vi "Calibracion.vi"() -> ()   [LabVIEW 2013]
uses:
  Multicard III_Hardware_Module Control.ctl
  P2022 TB INCAR GLOBALES.vi
panel:
  out "Waveform Chart":dbl(graph)
  in  "BorraGrafica":bool
  out "Estado":bool
  out "error out":errorcluster
  in  "error in (no error)":errorcluster
  out "Peso de calibración":string
  out "Lectura A/D ?":i32
  out "Termopar":string
  in  "CambioNP":bool
  out "Núm. promedios":i32 max=255 step=1
  out "Lectura A/D Cero":i32
  out "Lectura A/D Span":i32
  out "Lectura A/D":i32
  in  "Help":bool
  out "Peso (mg)":dbl format="%.3f"
  in  "Exit":bool
  in  "Calibrate":bool
  in  "Zero":bool
  out "Temperatura (C)":dbl format="%.1f"
  # "Calibración termobalanza"
  # "Termobalanza"
  # "Lecturas de calibración A/D"
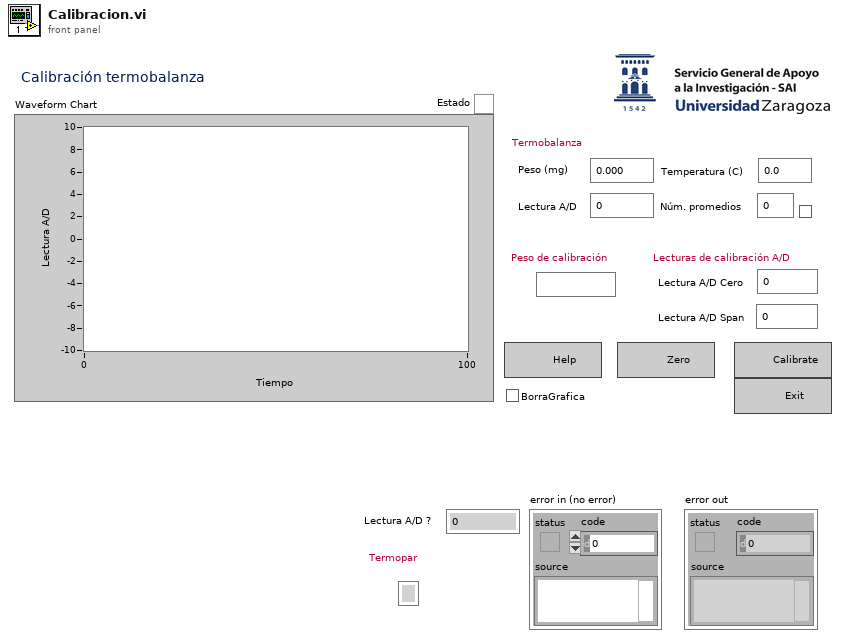
[diagram p1: front panel]
types:
  T1 = typedef "P2018 Com Control.ctl" = cluster{"Flujo_1":refnum<visa-resource-name>, "Brk1":bool, "Flujo_2":refnum<visa-resource-name>, "Brk2":bool, "Flujo_3":refnum<visa-resource-name>, "Brk3":bool, "Flujo_4":refnum<visa-resource-name>, "Brk4":bool, "Eurothe":refnum<visa-resource-name>, "Eurot":bool, "Balanza":refnum<visa-resource-name>, "Bal":bool, "eValPos":refnum<visa-resource-name>, "eVal":bool, "flowbus":refnum<visa-resource-name>, "fb":bool}
  T2 = typedef "Multicard III_Hardware_Module Control.ctl" = enum16{"Initialize", "Cero", "Span", "Read ugr", "Read mgr", "Read A/D", "Read T", "Number readings", "Thermocouple type", "Status", "Shutdown"}
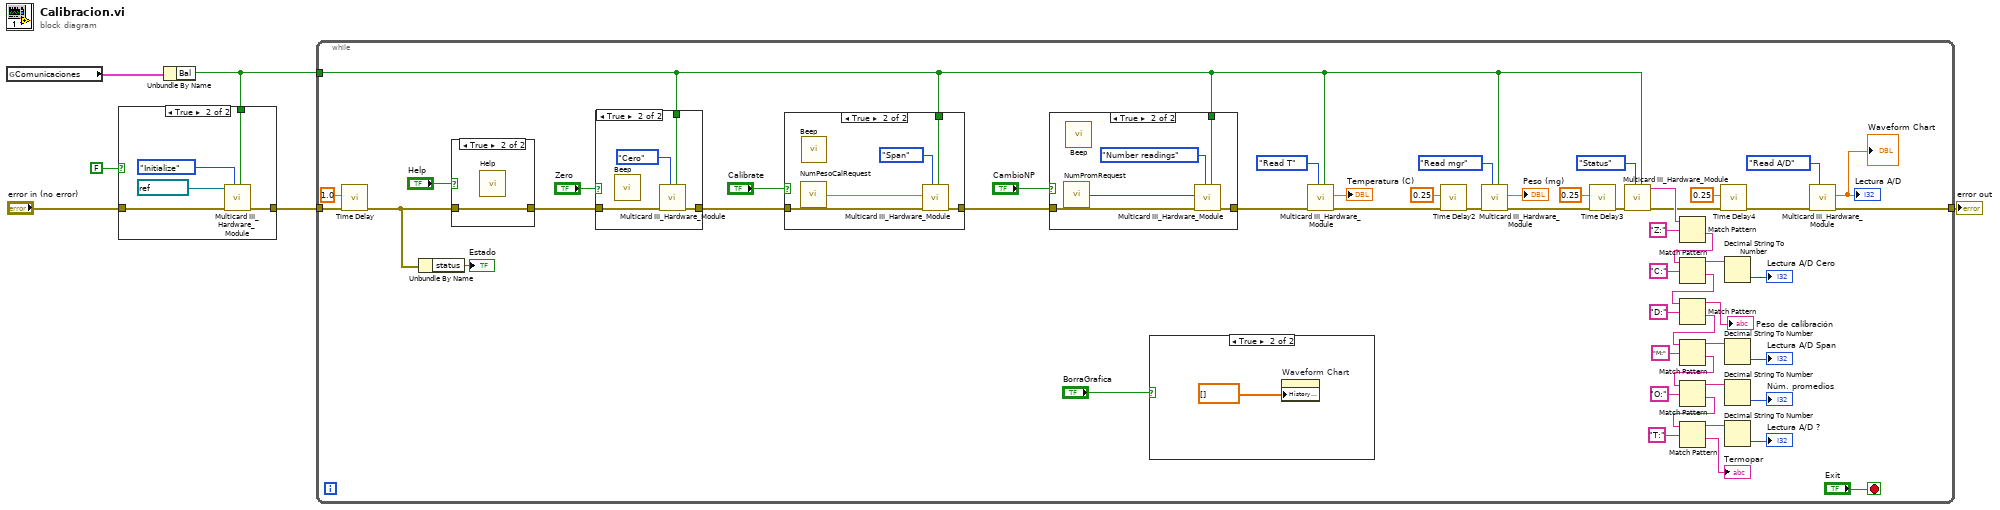
[diagram p0: block diagram]
diagram:
  n1 = global read "P2022 TB INCAR GLOBALES.vi" "Comunicaciones"() -> (w2:T1)
  n2 = Unbundle By Name(w2) -> ("Bal"=w1:bool)
  n3 = case shown="True" FALSE {
    tunnel: "error in (no error)" -> [w7 w11]
    tunnel: [w7 w10] -> w4
    tunnel: w1 -> [_ w8]
    frame False {
    }
    frame True {
      n4 = call "Multicard III_Hardware_Module.vi"("Multicard (T:Enable)"=w8, "Command"=Multicard_III_Hardware_Module_Control."Initialize", "error in (no error)"=w11, "VISA resource name"=refnum<visa-resource-name> "COM4") -> ("error out"=w10:errorcluster)  [unwired: 4 in, 3 out]
    }
  }
  n5 = while {
    tunnel: [w36] -> w6
    tunnel: w4 -> [w27]
    tunnel: w1 -> [w14]
    stop <- "Exit" stop-if-true
    n6 = call "Time Delay"("error in (no error)"=w27, "Delay Time (s)"=1.0) -> ("error out"=w26:errorcluster)  [unwired: 9 in]
    n7 = Unbundle By Name(w26) -> ("status"=→"Estado":bool)
    n8 = case shown="True" "Help" {
      tunnel: w26 -> [w80 w81]
      tunnel: [w80 w81] -> w35
      frame False {
      }
      frame True {
        n9 = call "Help.vi"() -> ()  [unwired: 1 in]
      }
    }
    n10 = case shown="True" "Zero" {
      tunnel: w35 -> [w82 w85]
      tunnel: [w82 w84] -> w33
      tunnel: w14 -> [_ w83]
      frame False {
      }
      frame True {
        n11 = call <vilib>:"Beep.vi"() -> ()  [unwired: 12 in]
        n12 = call "Multicard III_Hardware_Module.vi"("Multicard (T:Enable)"=w83, "Command"=Multicard_III_Hardware_Module_Control."Cero", "error in (no error)"=w85) -> ("error out"=w84:errorcluster)  [unwired: 5 in, 3 out]
      }
    }
    n13 = case shown="True" "Calibrate" {
      tunnel: w33 -> [w74 w76]
      tunnel: [w74 w78] -> w31
      tunnel: w14 -> [_ w75]
      frame False {
      }
      frame True {
        n14 = call "NumPesoCalRequest.vi"() -> ("NumProm"=w77:dbl)  [unwired: 1 in]
        n15 = call <vilib>:"Beep.vi"() -> ()  [unwired: 12 in]
        n16 = call "Multicard III_Hardware_Module.vi"("Multicard (T:Enable)"=w75, "Command"=Multicard_III_Hardware_Module_Control."Span", "error in (no error)"=w76, "Input Value"=w77) -> ("error out"=w78:errorcluster)  [unwired: 4 in, 3 out]
      }
    }
    n17 = case shown="True" "CambioNP" {
      tunnel: w31 -> [w68 w70]
      tunnel: [w68 w72] -> w30
      tunnel: w14 -> [_ w69]
      frame False {
      }
      frame True {
        n18 = call "NumPromRequest.vi"() -> ("NumProm"=w71:u8)  [unwired: 1 in]
        n19 = call <vilib>:"Beep.vi"() -> ()  [unwired: 12 in]
        n20 = call "Multicard III_Hardware_Module.vi"("Multicard (T:Enable)"=w69, "Command"=Multicard_III_Hardware_Module_Control."Number readings", "error in (no error)"=w70, "Input Value"=w71) -> ("error out"=w72:errorcluster)  [unwired: 4 in, 3 out]
      }
    }
    n21 = case shown="True" "BorraGrafica" {
      frame False {
      }
      frame True {
        n22 = property on="Waveform Chart" class="WFChart (strict)"("History Data"=dbl[] []) -> ()  [unwired: 2 in, 2 out]
      }
    }
    n23 = call "Multicard III_Hardware_Module.vi"("Multicard (T:Enable)"=w14, "Command"=Multicard_III_Hardware_Module_Control."Read T", "error in (no error)"=w30) -> ("error out"=w25:errorcluster, "Output Value"=→"Temperatura (C)":dbl)  [unwired: 5 in, 2 out]
    n24 = call "Time Delay2"("error in (no error)"=w25, "Delay Time (s)"=0.25) -> ("error out"=w24:errorcluster)  [unwired: 9 in]
    n25 = call "Multicard III_Hardware_Module.vi"("Multicard (T:Enable)"=w14, "Command"=Multicard_III_Hardware_Module_Control."Read mgr", "error in (no error)"=w24) -> ("error out"=w23:errorcluster, "Output Value"=→"Peso (mg)":dbl)  [unwired: 5 in, 2 out]
    n26 = call "Time Delay3"("error in (no error)"=w23, "Delay Time (s)"=0.25) -> ("error out"=w22:errorcluster)  [unwired: 9 in]
    n27 = call "Multicard III_Hardware_Module.vi"("Multicard (T:Enable)"=w14, "Command"=Multicard_III_Hardware_Module_Control."Status", "error in (no error)"=w22) -> ("error out"=w16:errorcluster, "String"=w39:string)  [unwired: 5 in, 2 out]
    n28 = Match Pattern(string=w39, regular expression="Z:") -> (after substring=w49:string)  [unwired: 1 in, 3 out]
    n29 = Match Pattern(string=w49, regular expression="C:") -> (before substring=w51:string, after substring=w48:string)  [unwired: 1 in, 2 out]
    n30 = Match Pattern(string=w48, regular expression="D:") -> (before substring=→"Peso de calibración":string, after substring=w50:string)  [unwired: 1 in, 2 out]
    n31 = Match Pattern(string=w50, regular expression="M:") -> (before substring=w52:string, after substring=w44:string)  [unwired: 1 in, 2 out]
    n32 = Match Pattern(string=w44, regular expression="O:") -> (before substring=w53:string, after substring=w43:string)  [unwired: 1 in, 2 out]
    n33 = Match Pattern(string=w43, regular expression="T:") -> (before substring=w54:string, after substring=→"Termopar":string)  [unwired: 1 in, 2 out]
    n34 = call "Time Delay4"("error in (no error)"=w16, "Delay Time (s)"=0.25) -> ("error out"=w15:errorcluster)  [unwired: 9 in]
    n35 = Decimal String To Number(string=w51) -> (number=→"Lectura A/D Cero":i32)  [unwired: 2 in, 1 out]
    n36 = Decimal String To Number(string=w52) -> (number=→"Lectura A/D Span":i32)  [unwired: 2 in, 1 out]
    n37 = Decimal String To Number(string=w53) -> (number=→"Núm. promedios":i32)  [unwired: 2 in, 1 out]
    n38 = Decimal String To Number(string=w54) -> (number=→"Lectura A/D ?":i32)  [unwired: 2 in, 1 out]
    n39 = call "Multicard III_Hardware_Module.vi"("Command"=Multicard_III_Hardware_Module_Control."Read A/D", "error in (no error)"=w15) -> ("error out"=w36:errorcluster, "Output Value"=→"Lectura A/D" →"Waveform Chart":dbl)  [unwired: 6 in, 2 out]
  }
  "error out" <- w6
